vi "FileExplore.vi"() -> ()   [LabVIEW 2011]
panel:
  in  "Multicolumn Listbox":i32(listbox)
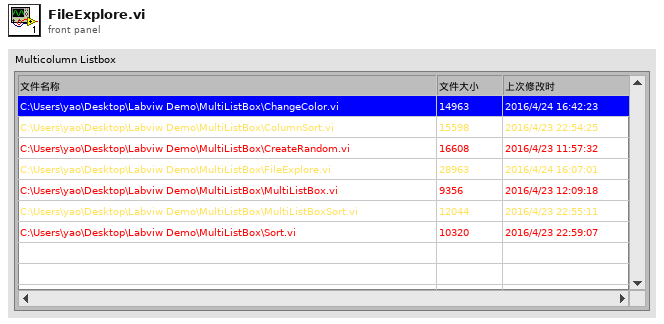
[diagram p1: front panel]
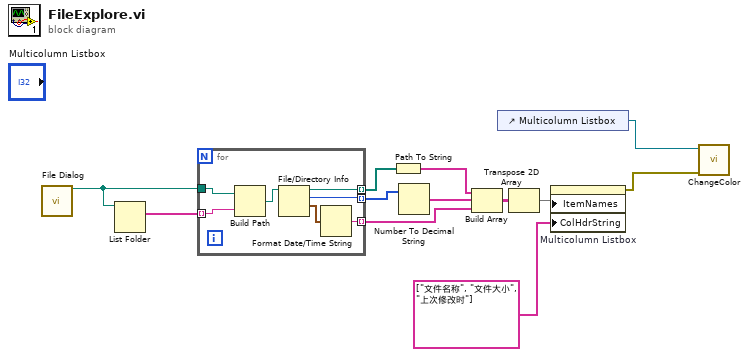
[diagram p0: block diagram]
diagram:
  n1 = call "File Dialog"() -> ("selected path"=w12:path)  [unwired: 12 in, 3 out]
  n2 = List Folder(path=w12) -> (filenames=w11:string[])  [unwired: 3 in, 3 out]
  n3 = for {
    tunnel: w12 -> [w18]
    tunnel: w11 -> [w17] mode=indexing
    tunnel: [w16] -> w10 mode=indexing
    tunnel: [w15] -> w9 mode=indexing
    tunnel: [w13] -> w6 mode=indexing
    n4 = Build Path(base path=w18, name or relative path=w17) -> (appended path=w19:path)
    n5 = File/Directory Info(path=w19) -> (path out=w16:path, size=w15:i64, last mod=w14:timestamp)  [unwired: 1 in, 4 out]
    n6 = Format Date/Time String(seconds (now)=w14) -> (date/time string=w13:string)  [unwired: 2 in]
  }
  n7 = Path To String(path=w10) -> (string=w8:string[])
  n8 = Number To Decimal String(number=w9) -> (decimal integer string=w7:string[])  [unwired: 1 in]
  n9 = Build Array(w8, w7, w6) -> (w5:string[][])
  n10 = control-ref of="Multicolumn Listbox"() -> (w1:refnum<vi>)
  n11 = Transpose 2D Array(2D array=w5) -> (transposed array=w3:string[][])
  n12 = property on="Multicolumn Listbox" class="MCListbox (strict)"("ItemNames"=w3, "ColHdrString"=string[] ["文件名称", "文件大小", "上次修改时"] ("Column Header Strings[]")) -> (error out=w2:errorcluster)  [unwired: 2 in, 1 out]
  n13 = call "ChangeColor.vi"("error in (no error)"=w2, "MCListbox Refnum"=w1) -> ()  [unwired: 9 in, 1 out]
